vi "Begin.vi"(8 "error in":errorcluster) -> (0 "error out":errorcluster)   [LabVIEW 2019]
doc: "Called before other user functions, this VI is expected to open initial I/O refnums, load in file data, and do all program initialization. Notice that the <B>error out</B> terminal is simply used for data flow. Wiring it to other structures or subVIs ensures that this VI runs first."
uses:
  <vilib>/Rock Robotics/WPI/DriverStation/WPI_DriverStationRobotMode2.ctl
  <vilib>/Rock Robotics/WPI/Joystick/WPI_JoystickDeviceEnum.ctl
  Robot Global Data.vi
  <vilib>/Rock Robotics/Network Tables/NT Write String Array.vi
  <vilib>/Rock Robotics/WPI/ThirdParty/Phoenix-LabVIEW/CANCoder/Controls/CTRE_Phoenix_CANcoder_SensorInitializationStrategy.ctl
  <vilib>/Rock Robotics/WPI/ThirdParty/Phoenix-LabVIEW/CANCoder/Controls/CTRE_Phoenix_CANcoder_AbsoluteSensorRange.ctl
  <vilib>/Rock Robotics/WPI/ThirdParty/Phoenix-LabVIEW/CANCoder/Controls/CTRE_Phoenix_CANcoder_SensorTimeBase.ctl
  <vilib>/Rock Robotics/WPI/ThirdParty/Phoenix-LabVIEW/Motor Controller/Controls/CTRE_Phoenix_MotorControl_VelocityMeasurementPeriod.ctl
  <vilib>/Rock Robotics/WPI/ThirdParty/Phoenix-LabVIEW/CANCoder/Controls/CTRE_Phoenix_CANcoder_Configurables.ctl
panel:
  in  "CANcoder Configurables":T1={"Sensor Initialization Strategy"=enum."Boot To Zero", "Absolute Sensor Range"=enum."Signed [-180 to +180)", "Velocity Measurement Period"=100, "Velocity Measurement Window"=64, "Magnet Offset (Degrees)"=0.0, "Sensor Direction"=FALSE, "Sensor Coefficient"=0.087890625, "Unit String"="penguins!", "Sensor Time Base"=enum."PerMinute"} {"Velocity Measurement Period" items=["Period_1ms"=1, "Period_2ms"=2, "Period_5ms"=5, "Period_10ms"=10, "Period_20ms"=20, "Period_25ms"=25, "Period_50ms"=50, "Period_100ms"=100]; "Sensor Coefficient" format="%#_9g"}
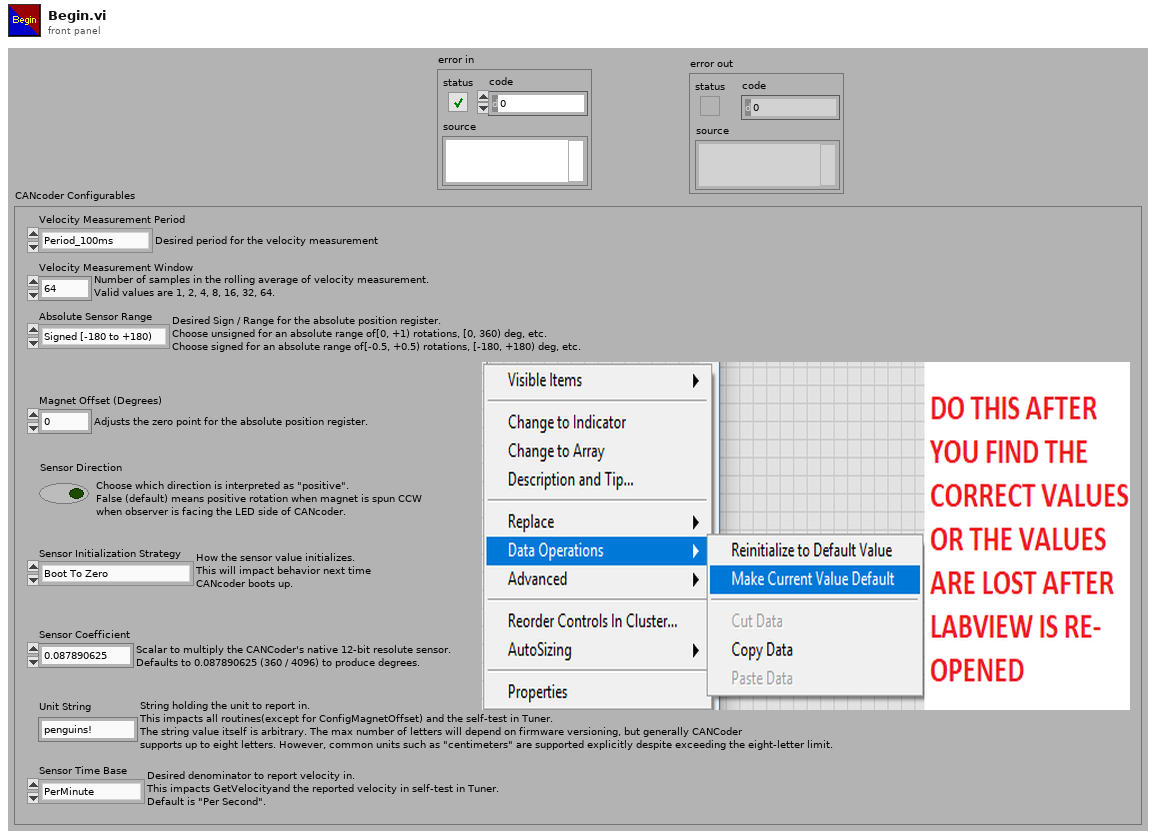
[diagram p1: front panel]
types:
  T1 = typedef "CTRE_Phoenix_CANcoder_Configurables.ctl" = cluster{"Sensor Initialization Strategy":T2, "Absolute Sensor Range":T3, "Velocity Measurement Period":T4, "Velocity Measurement Window":i32, "Magnet Offset (Degrees)":dbl, "Sensor Direction":bool, "Sensor Coefficient":dbl, "Unit String":string, "Sensor Time Base":T5}
  T2 = typedef "CTRE_Phoenix_CANcoder_SensorInitializationStrategy.ctl" = enum16{"Boot To Zero", "Boot To Absolute Position"}
  T3 = typedef "CTRE_Phoenix_CANcoder_AbsoluteSensorRange.ctl" = enum16{"Unsigned [0 to 360)", "Signed [-180 to +180)"}
  T4 = typedef "CTRE_Phoenix_MotorControl_VelocityMeasurementPeriod.ctl" = u16
  T5 = typedef "CTRE_Phoenix_CANcoder_SensorTimeBase.ctl" = enum16{"Per100Ms_Legacy", "PerSecond", "PerMinute"}
  T6 = typedef "WPI_JoystickDeviceEnum.ctl" = enum16{"USB 0", "USB 1", "USB 2", "USB 3", "USB 4", "USB 5"}
  T7 = typedef "WPI_DriverStationRobotMode2.ctl" = enum16{"Autonomous Disabled", "Autonomous Enabled", "Teleop Disabled", "Teleop Enabled", "Disconnected", "Finish", "Test Disabled", "Test Enabled", "Emergency Stopped"}
  T8 = typedef "WPI_JoystickDevRef.ctl" = cluster{"Device":T6}
  T9 = typedef "CTRE_Phoenix_CANcoder_DeviceRef.ctl" = cluster{"DeviceStatus":errorcluster, "Device Number":u8, "Handle":u64, "UsageFrame":u32, "Library Path":path}
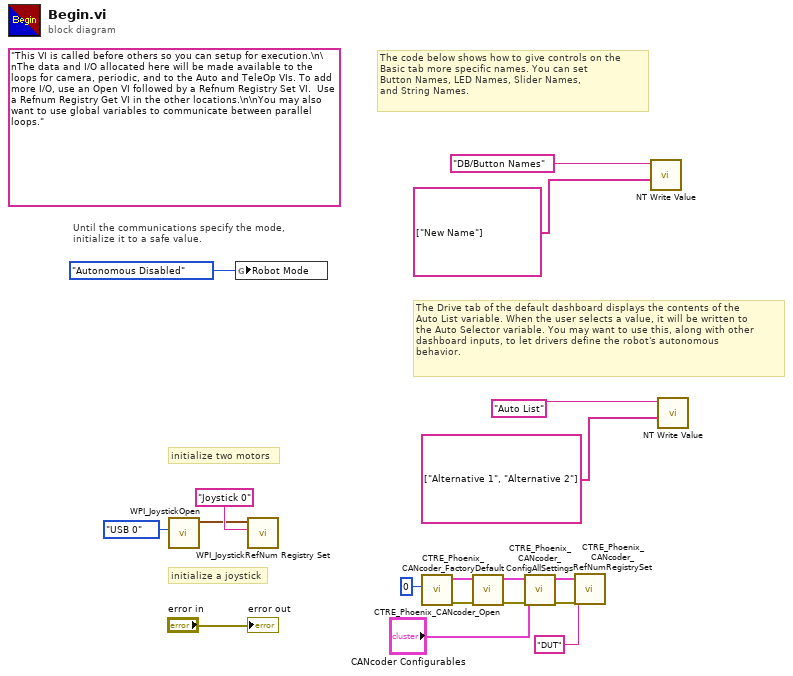
[diagram p0: block diagram]
diagram:
  (unwired) "This VI is called before others so you can setup for execution.\n\nThe data and I/O allocated here will be made available to the loops for camera, periodic, and to the Auto and TeleOp VIs. To add more I/O, use an Open VI followed by a Refnum Registry Set VI.  Use a Refnum Registry Get VI in the other locations.\n\nYou may also want to use global variables to communicate between parallel loops."
  # "The Drive tab of the default dashboard displays the contents of the\nAuto List variable. When the user selects a value, it will be written to\nthe Auto Selector variable. You may want to use this, along with other\ndashboard inputs, to let drivers define the robot's autonomous\nbehavior."
  # "The code below shows how to give controls on the\nBasic tab more specific names. You can set\nButton Names, LED Names, Slider Names,\nand String Names."
  # "initialize a joystick"
  # "Until the communications specify the mode,\ninitialize it to a safe value."
  # "initialize two motors"
  n1 = call <vilib>:"WPI_JoystickOpen.vi"("JoystickDevice"=WPI_JoystickDeviceEnum."USB 0") -> ("JoystickDevRef"=w16:T8)  [unwired: 10 in]
  n2 = global write "Robot Global Data.vi" "Robot Mode"(WPI_DriverStationRobotMode2."Autonomous Disabled" ("Robot Mode")) -> ()
  n3 = call <vilib>:"WPI_JoystickRefNum Registry Set.vi"("refnum name"="Joystick 0", "JoystickDevRef"=w16) -> ()  [unwired: 8 in, 2 out]
  n4 = call <vilib>:"CTRE_Phoenix_CANcoder_Open.vi"("Device Number"=u8 0) -> ("error out"=w8:errorcluster, "CTRE_CANcoder_DeviceRef"=w7:T9)  [unwired: 9 in]
  n5 = call <vilib>:"CTRE_Phoenix_CANcoder_FactoryDefault.vi"("error in"=w8, "CTRE_CANcoder_DeviceRef"=w7) -> ("error out"=w6:errorcluster, "CTRE_CANcoder_DeviceRef"=w5:T9)  [unwired: 8 in]
  n6 = call <vilib>:"CTRE_Phoenix_CANcoder_ConfigAllSettings.vi"("error in (no error)"=w6, "CANcoder Configurables"="CANcoder Configurables", "CTRE_CANcoder_DeviceRef"=w5) -> ("error out"=w3:errorcluster, "CTRE_CANcoder_DeviceRef"=w2:T9)  [unwired: 7 in]
  n7 = call <vilib>:"CTRE_Phoenix_CANcoder_RefNumRegistrySet.vi"("error in (no error)"=w3, "refnum name"="DUT", "CTRE_CANcoder_DeviceRef"=w2) -> ()  [unwired: 7 in, 2 out]
  n8 = call-poly <vilib>:"NT Write Value.vi"("String Array"=string[] ["New Name"], "Name"="DB/Button Names") -> ()  [unwired: 9 in, 1 out]
  n9 = call-poly <vilib>:"NT Write Value.vi"("String Array"=string[] ["Alternative 1", "Alternative 2"], "Name"="Auto List") -> ()  [unwired: 9 in, 1 out]
  "error out" <- "error in"
